vi "Actor Core.vi"(8 "error in":errorcluster, 11 "TimerViewSmall in":refnum<class "TimerViewSmall.lvclass">) -> (0 "error out":errorcluster, 3 "Actor out":refnum<class "Actor.lvclass">)   [LabVIEW 2012, in "TimerSensor.lvlib" / "TimerViewSmall.lvclass"]
doc: "(<B>Filename</B>: Actor Framework.lvlib:Actor.lvclass:Actor Core.vi)\n\nReceives messages to the actor, reacts to them, and initiates any error handling that may shut the actor down.\n\nDescendant classes may override this VI to append parallel tasks for the actor to complete while it handles messages. Overrides use the Call Parent Method node."
uses:
  TimerViewSmall.lvclass
  <vilib>/ActorFramework/Actor/Actor.lvclass
  Sensor Definition/SensorViewSmall.lvclass
  <vilib>/ActorFramework/Actor/Actor.lvclass/Actor.ctl
  Win8uiFramework/ViewableActor.lvclass/ViewableActor.ctl
  Sensor Definition/SensorView.lvclass/SensorView.ctl
  TimerSensorConfig.lvclass
  Sensor Definition/SensorInfo.lvclass/SensorInfo.ctl
  TimerSensorConfig.lvclass/TimerSensorConfig.ctl
  Sensor Definition/Double Scalar SensorData.lvclass
  <vilib>/ActorFramework/Message Enqueuer/Message Enqueuer.lvclass/Message Enqueuer.ctl
  Sensor Definition/SensorInfo/Read Name.vi
  Sensor Definition/SensorInfo/Read Description.vi
  Sensor Definition/Read Config.vi
  TimerSensorConfig/Read Target Time.vi
  TimerSensorConfig/Read Timer Direction.vi
  Win8uiFramework/Read Stop Event.vi
  Sensor Definition/SensorView/Read SensorInfo Changed Event.vi
  Sensor Definition/SensorView/Read SensorData Changed Event.vi
  <vilib>/ActorFramework/Message Enqueuer/Enqueue.vi
  <vilib>/ActorFramework/Message Priority Queue/Priority Enqueue.vi
  <vilib>/Utility/cursorutil.llb/Set Cursor (Icon Pict).vi
  Sensor Definition/SensorInfo.lvclass
  Sensor Definition/SensorData.lvclass
  Sensor Definition/SensorConfig.lvclass
  Sensor Messages/Launch Detail View Msg/Launch Detail View Msg.lvclass
  Win8uiFramework/ViewableActor.lvclass
panel:
  in  "Centered String Hack":bool
  out "Title":string="Application Title"
  out "Target Time":timestamp format="%<%I:%M:%S %p\n%m/%d/%Y>T"
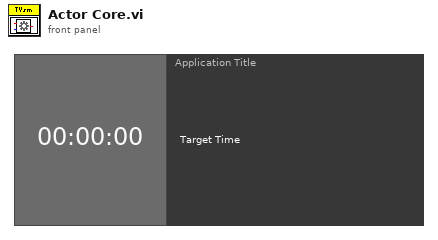
[diagram p1: front panel]
types:
  T1 = typedef "Timer Direction.ctl" = enum16{"Up", "Down"}
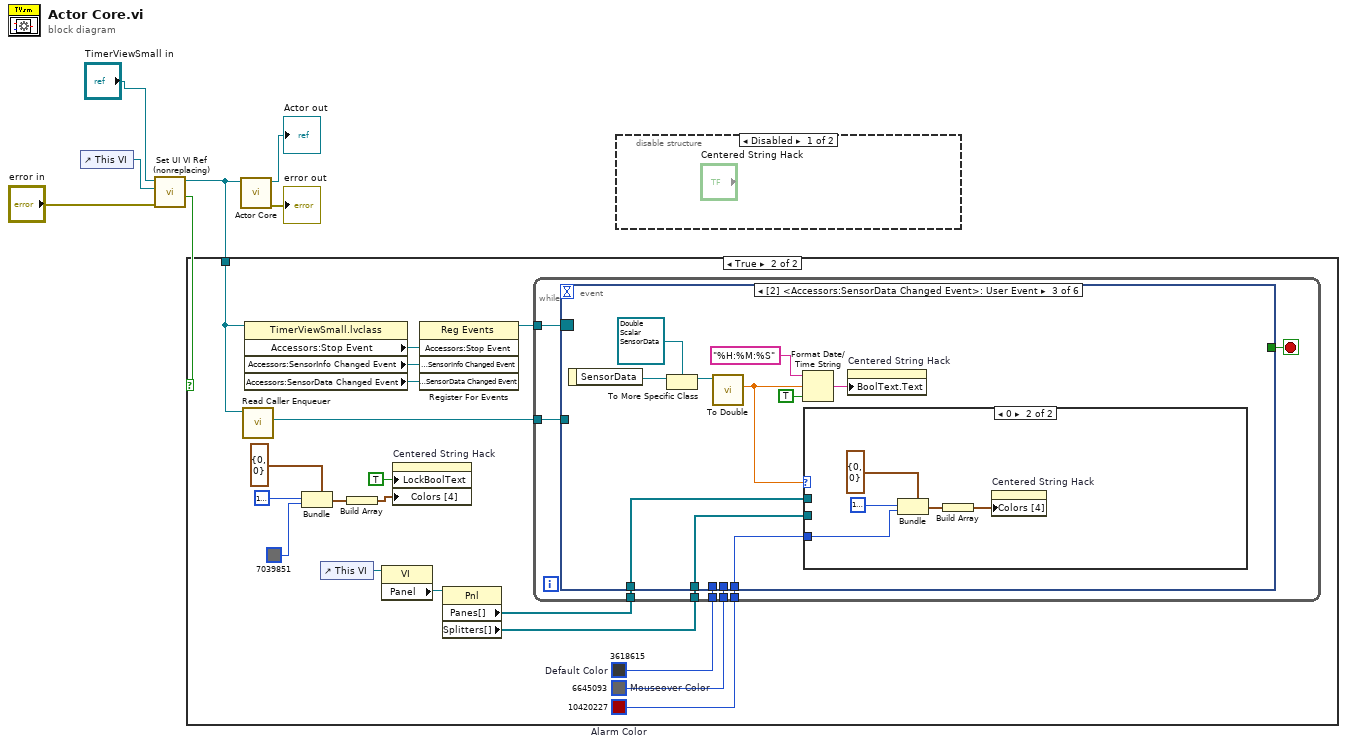
[diagram p0: block diagram]
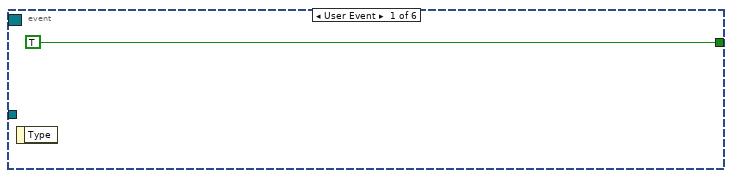
[diagram p4: hidden frame]
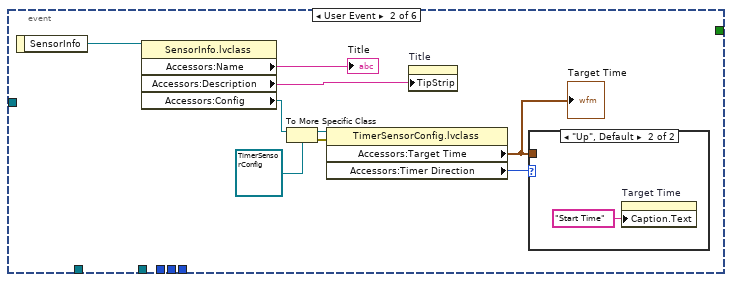
[diagram p5: hidden frame]
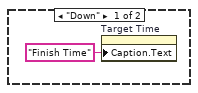
[diagram p6: hidden frame]
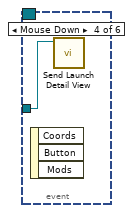
[diagram p8: hidden frame]
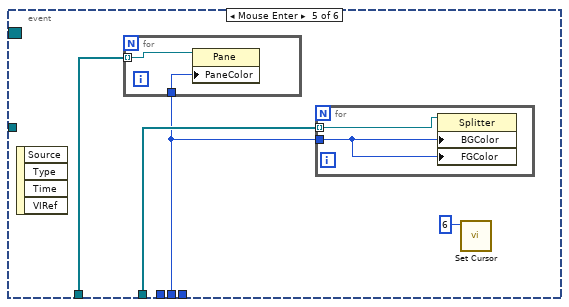
[diagram p9: hidden frame]
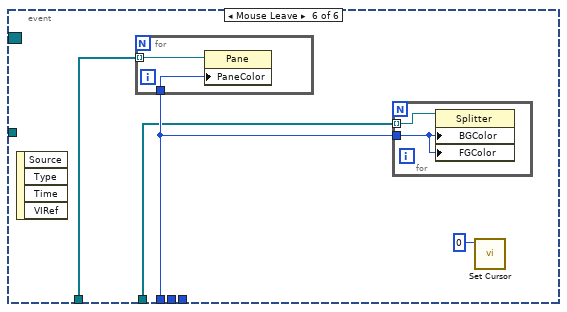
[diagram p10: hidden frame]
diagram:
  n1 = control-ref of="This VI"() -> (w5:refnum<vi>)
  n2 = call "Set UI VI Ref (nonreplacing).vi"("error in (no error)"="error in", "UI VI Ref"=w5, "ViewableActor in"="TimerViewSmall in") -> ("Top Level UI?"=w1:bool, "ViewableActor out"=w2:refnum<class "TimerViewSmall.lvclass">)  [unwired: 6 in, 1 out]
  n3 = case shown="True" w1 {
    tunnel: w2 -> [_ w22]
    frame False {
    }
    frame True {
      w13 = u32 10420227  # Alarm Color
      w20 = u32 6645093  # Mouseover Color
      w19 = u32 3618615  # Default Color
      n4 = call <vilib>:"Read Caller Enqueuer.vi"("Actor"=w22) -> ("Caller Enqueuer"=w21:refnum<class "Message Enqueuer.lvclass">)  [unwired: 10 in]
      n5 = property class="TimerViewSmall.lvclass"(reference=w22) -> ("Accessors:Stop Event"=w26:refnum<user-event>, "Accessors:SensorInfo Changed Event"=w25:refnum<user-event>, "Accessors:SensorData Changed Event"=w23:refnum<user-event>)  [unwired: 1 in, 2 out]
      n6 = Bundle(cluster=cluster{u32, u32} {0, 0}, u32 16777216 ("Default Color"), u32 7039851 ("Default Color")) -> (w11:cluster{u32, u32})
      n7 = control-ref of="This VI"() -> (w18:refnum<vi>)
      n8 = Build Array(w11) -> (w9:cluster{u32, u32}[])
      n9 = property class="VI"(reference=w18) -> ("Panel"=w17:refnum<vi>)  [unwired: 1 in, 2 out]
      n10 = property on="Centered String Hack" class="Bool (strict)"("LockBoolText"=TRUE ("Lock Boolean Text In Center"), "Colors [4]"=w9) -> ()  [unwired: 2 in, 2 out]
      n11 = register-events(w26, w25, w23) -> (reference out=w24:refnum<event-registration>)  [unwired: 2 in, 1 out]
      n12 = property class="Pnl"(reference=w17) -> ("Panes[]"=w16:refnum<vi>[], "Splitters[]"=w15:refnum<vi>[])  [unwired: 1 in, 2 out]
      n13 = while {
        tunnel: w24 -> [w34]
        tunnel: w21 -> [w32]
        tunnel: w16 -> [w31]
        tunnel: w20 -> [w30]
        tunnel: w19 -> [w29]
        tunnel: w15 -> [w28]
        tunnel: w13 -> [w27]
        stop <- w33 stop-if-true
        n14 = event shown="[2] <Accessors:SensorData Changed Event>: User Event" {
          selector: w34 -> [_ _ _ _ _ _]
          dyn-events: _ -> [_ _ _ _ _ _]
          timeout: _ -> [_ _ _ _ _ _]
          tunnel: [TRUE _ _ _ _ _] -> w33
          tunnel: w32 -> [_ _ _ w62 _ _]
          tunnel: w31 -> [_ _ w49 _ w66 w74]
          tunnel: w30 -> [_ _ _ _ w64 _]
          tunnel: w29 -> [_ _ _ _ _ w73]
          tunnel: w28 -> [_ _ w48 _ w65 w72]
          tunnel: w27 -> [_ _ w47 _ _ _]
          event User Event {
            n15 = event-data() -> ()  [unwired: 1 in, 1 out]
          }
          event User Event {
            n16 = event-data() -> ("SensorInfo"=w42:refnum<class "SensorInfo.lvclass">)  [unwired: 1 in]
            n17 = property class="SensorInfo.lvclass"(reference=w42) -> ("Accessors:Name"=→"Title":string, "Accessors:Description"=w43:string, "Accessors:Config"=w41:refnum<class "SensorConfig.lvclass">)  [unwired: 1 in, 2 out]
            n18 = To More Specific Class(target class=refnum<class "TimerSensorConfig.lvclass"> refnum ("TimerSensor.lvlib:TimerSensorConfig.lvclass"), reference=w41) -> (specific class reference=w38:refnum<class "TimerSensorConfig.lvclass">, error out=w39:errorcluster)  [unwired: 1 in]
            n19 = property class="TimerSensorConfig.lvclass"(reference=w38, error in=w39) -> ("Accessors:Target Time"=w37:timestamp, "Accessors:Timer Direction"=w36:T1)  [unwired: 2 out]
            "Target Time" <- w37
            n20 = property on="Title" class="Str"("TipStrip"=w43) -> ()  [unwired: 2 in, 2 out]
            n21 = case shown="\"Up\", Default" w36 {
              tunnel: w37 -> [_ _]
              frame "Down" {
                n22 = property on="Target Time" class="AbsTime (strict)"("Caption.Text"="Finish Time" ("Label.Text")) -> ()  [unwired: 2 in, 2 out]
              }
              frame "Up", Default {
                n23 = property on="Target Time" class="AbsTime (strict)"("Caption.Text"="Start Time" ("Label.Text")) -> ()  [unwired: 2 in, 2 out]
              }
            }
          }
          event User Event {
            n24 = event-data() -> ("SensorData"=w56:refnum<class "SensorData.lvclass">)  [unwired: 1 in]
            n25 = To More Specific Class(target class=refnum<class "Double Scalar SensorData.lvclass"> refnum ("Sensor Definition.lvlib:Double Scalar SensorData.lvclass"), reference=w56) -> (specific class reference=w55:refnum<class "Double Scalar SensorData.lvclass">)  [unwired: 1 in, 1 out]
            n26 = call-dynamic "To Double.vi"("Double Scalar SensorData in"=w55) -> ("Value"=w50:dbl)  [unwired: 8 in, 2 out]
            n27 = Format Date/Time String(time format string (%c)="%H:%M:%S", seconds (now)=w50, UTC format=TRUE) -> (date/time string=w51:string)
            n28 = case shown="0" w50 {
              tunnel: w49 -> [_ _]
              tunnel: w48 -> [_ _]
              tunnel: w47 -> [_ w60]
              frame Default {
              }
              frame 0 {
                n29 = Bundle(cluster=cluster{u32, u32} {0, 0}, u32 16777216 ("Default Color"), w60) -> (w59:cluster{u32, u32})
                n30 = Build Array(w59) -> (w58:cluster{u32, u32}[])
                n31 = property on="Centered String Hack" class="Bool (strict)"("Colors [4]"=w58) -> ()  [unwired: 2 in, 2 out]
              }
            }
            n32 = property on="Centered String Hack" class="Bool (strict)"("BoolText.Text"=w51) -> ()  [unwired: 2 in, 2 out]
          }
          event Mouse Down {
            n33 = event-data() -> ()  [unwired: 1 in, 3 out]
            n34 = call "Send Launch Detail View.vi"("Message Enqueuer"=w62) -> ()  [unwired: 9 in, 2 out]
          }
          event Mouse Enter {
            n35 = event-data() -> ()  [unwired: 1 in, 4 out]
            n36 = for {
              tunnel: w66 -> [w69] mode=indexing
              tunnel: w64 -> [w70]
              n37 = property class="Pane"(reference=w69, "PaneColor"=w70) -> ()  [unwired: 1 in, 2 out]
            }
            n38 = for {
              tunnel: w65 -> [w67] mode=indexing
              tunnel: w64 -> [w68]
              n39 = property class="Splitter"(reference=w67, "BGColor"=w68, "FGColor"=w68) -> ()  [unwired: 1 in, 2 out]
            }
            n40 = call-poly <vilib>:"Set Cursor.vi"("icon"=u16 6) -> ()  [unwired: 9 in, 2 out]
          }
          event Mouse Leave {
            n41 = event-data() -> ()  [unwired: 1 in, 4 out]
            n42 = for {
              tunnel: w74 -> [w77] mode=indexing
              tunnel: w73 -> [w78]
              n43 = property class="Pane"(reference=w77, "PaneColor"=w78) -> ()  [unwired: 1 in, 2 out]
            }
            n44 = for {
              tunnel: w72 -> [w75] mode=indexing
              tunnel: w73 -> [w76]
              n45 = property class="Splitter"(reference=w75, "BGColor"=w76, "FGColor"=w76) -> ()  [unwired: 1 in, 2 out]
            }
            n46 = call-poly <vilib>:"Set Cursor.vi"("icon"=u16 0) -> ()  [unwired: 9 in, 2 out]
          }
        }
      }
    }
  }
  n47 = call-parent "Actor Core.vi"("SensorViewSmall in"=w2) -> ("error out"=→"error out":errorcluster, "Actor out"=→"Actor out":refnum<class "Actor.lvclass">)  [unwired: 9 in]
  n48 = disable-structure shown="Disabled" {
    frame Disabled {
    }
    frame Enabled {
    }
  }
